vi "img test 11(calibration).vi"(7 "error in":errorcluster) -> (27 "error out":errorcluster)   [LabVIEW 2009]
uses:
  <vilib>/vision/NI_Vision_Development_Module.lvlib
panel:
  out "Image Out":T1(plugin-control)
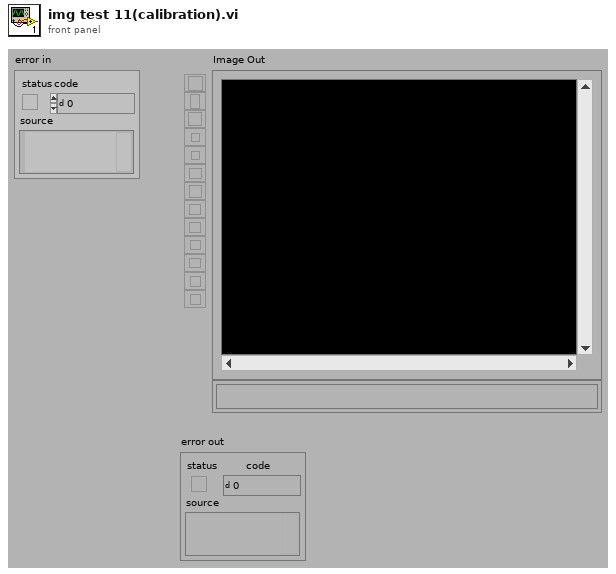
[diagram p1: front panel]
types:
  T1 = typedef "IMAQ Image.ctl" = refnum<image>
  T2 = enum32{"AutoM", "Close", "Dilate", "Erode", "Gradient", "Gradient out", "Gradient in", "Hit miss", "Open", "PClose", "POpen", "Thick", "Thin"}
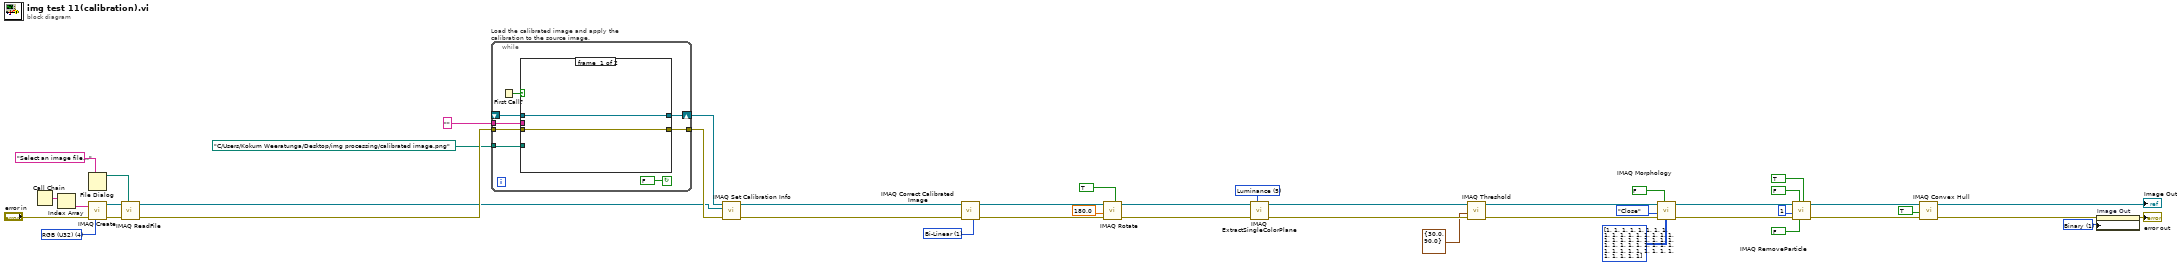
[diagram p0: block diagram]
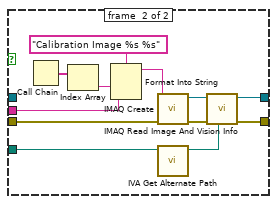
[diagram p2: hidden frame]
diagram:
  w2 = u32 1 items=["Grayscale", "Binary", "Gradient", "Rainbow", "Temperature", "User Defined"] ("Palette")
  w23 = 5 items=["Red", "Green", "Blue", "Hue", "Saturation", "Luminance", "Value", "Intensity"] ("Color Plane")
  w30 = u32 1 items=["Zero Order", "Bi-Linear", "Quadratic", "Cubic Spline"] ("Interpolation Type")
  w42 = u32 4 items=["Grayscale (U8)", "Grayscale (I16)", "Grayscale (SGL)", "Complex (CSG)", "RGB (U32)", "HSL (U32)", "RGB (U64)"] ("Image Type")
  n1 = Call Chain() -> (call chain=w38:string[])
  n2 = Index Array(array=w38) -> (element=w37:string)  [unwired: 1 in]
  n3 = File Dialog(7:"Select an image file..." ("prompt")) -> (3:w41:path)  [unwired: 1 in, 8 out]
  n4 = call "IMAQ Create"("Image Name"=w37, "Image Type"=w42, "error in (no error)"="error in") -> ("New Image"=w44:T1, "error out"=w43:errorcluster)  [unwired: 1 in, 1 out]
  n5 = call "IMAQ ReadFile"("File Path"=w41, "error in (no error)"=w43, "Image"=w44) -> ("error out"=w45:errorcluster, "Image Out"=w32:T1)  [unwired: 2 in, 5 out]
  n6 = while "Load the calibrated image and apply the calibration to the source image." {
    shift-right: [w52] -> w35
    shift-left: _ -> [w51]
    tunnel: [w49] -> w34
    tunnel: w45 -> [w48]
    tunnel: path "C:/Users/Kokum Weeratunga/Desktop/img processing/calibrated image.png" ("File Path") -> [w47]
    tunnel: "" ("Step Name") -> [w46]
    stop <- FALSE continue-if-true
    n7 = First Call?() -> (First Call?: T/F=w53:bool)
    n8 = case shown="True" w53 {
      tunnel: [w55 w65] -> w52
      tunnel: w51 -> [w55 _]
      tunnel: [w54 w62] -> w49
      tunnel: w48 -> [w54 w61]
      tunnel: w47 -> [_ w58]
      tunnel: w46 -> [_ w56]
      frame #0 {
      }
      frame #1 {
        n9 = Call Chain() -> (call chain=w60:string[])
        n10 = Index Array(array=w60) -> (element=w59:string)  [unwired: 1 in]
        n11 = Format Into String(format string="Calibration Image %s %s" ("Image Name"), w59, w56) -> (resulting string=w67:string)  [unwired: 2 in, 1 out]
        n12 = call "IMAQ Create"("Image Name"=w67, "error in (no error)"=w61) -> ("New Image"=w64:T1, "error out"=w63:errorcluster)  [unwired: 2 in, 1 out]
        n13 = call <vilib>:"IVA Get Alternate Path.vi"("Path In"=w58) -> ("Path Out"=w57:path)  [unwired: 10 out]
        n14 = call "IMAQ Read Image And Vision Info"("File Path"=w57, "error in (no error)"=w63, "Image"=w64) -> ("error out"=w62:errorcluster, "Image Out"=w65:T1)  [unwired: 1 in, 6 out]
      }
    }
  }
  n15 = call "IMAQ Set Calibration Info"("error in (no error)"=w34, "Image Dst"=w32, "Image Src"=w35) -> ("error out"=w33:errorcluster, "Calibrated Image"=w28:T1)  [unwired: 1 in, 6 out]
  n16 = call "IMAQ Correct Calibrated Image"("Interpolation Type"=w30, "error in (no error)"=w33, "Image Src"=w28) -> ("error out"=w29:errorcluster, "Corrected Image"=w27:T1)  [unwired: 4 in, 3 out]
  n17 = call "IMAQ Rotate"("Maintain Size"=TRUE, "error in (no error)"=w29, "Angle (degrees)"=sgl 180.0, "Image Src"=w27) -> ("error out"=w26:errorcluster, "Image Dst Out"=w22:T1)  [unwired: 4 in, 2 out]
  n18 = call "IMAQ ExtractSingleColorPlane"("Color Plane"=w23, "error in (no error)"=w26, "Image Src"=w22) -> ("error out"=w21:errorcluster, "Image Dst Out"=w19:T1)  [unwired: 1 in, 6 out]
  n19 = call "IMAQ Threshold"("error in (no error)"=w21, "Range"=cluster{"Lower value":sgl, "Upper value":sgl} {"Lower value"=30.0, "Upper value"=90.0}, "Image Src"=w19) -> ("error out"=w18:errorcluster, "Image Dst Out"=w14:T1)  [unwired: 3 in, 4 out]
  n20 = call "IMAQ Morphology"("Structuring Element"=i32[][] [[1, 1, 1, 1, 1, 1, 1], [1, 1, 1, 1, 1, 1, 1], [1, 1, 1, 1, 1, 1, 1], [1, 1, 1, 1, 1, 1, 1], [1, 1, 1, 1, 1, 1, 1], [1, 1, 1, 1, 1, 1, 1], [1, 1, 1, 1, 1, 1, 1]], "Square/Hexa (Square)"=FALSE, "error in (no error)"=w18, "Operation"=T2."Close", "Image Src"=w14) -> ("error out"=w13:errorcluster, "Image Dst Out"=w8:T1)  [unwired: 2 in, 3 out]
  n21 = call "IMAQ RemoveParticle"("Connectivity 4/8 (8)"=TRUE, "Low Pass/High Pass (Low)"=FALSE, "Square/Hexa (Square)"=FALSE, "error in (no error)"=w13, "Number of Erosion"=1, "Image Src"=w8) -> ("error out"=w7:errorcluster, "Image Dst Out"=w6:T1)  [unwired: 1 in, 3 out]
  n22 = call "IMAQ Convex Hull"("error in (no error)"=w7, "Connectivity 4/8 (8)"=TRUE, "Image Src"=w6) -> ("error out"=w4:errorcluster, "Image Dst Out"=→"Image Out":T1)  [unwired: 1 in, 6 out]
  n23 = property on="Image Out" class="ImageControl"(error in=w4, "Palette:Palette Type"=w2) -> (error out=→"error out":errorcluster)  [unwired: 1 in, 1 out]
